vi "231124_Nikon_Control.vi"() -> ()   [LabVIEW 2025]
doc: "This simple VI control few elements of a Nikon Ti2 microscope.\nAny kind of supplementary element can be controlled with a new event type (flurorescence cube turret for example)"
uses:
  v2.1/SubVIS/Presets.ctl
panel:
  in  "Presets":T1=2 items=["1- Bino - Brightfield"=1, "2- Bino - Fluo"=2, "3- Right"=3, "4- Left"=4]
  in  "Cluster commandes":T2={"Dia lamp"=TRUE, "Dia lamp intensity"=1689.1304347826087, "Objective"=2, "Light path"=2, "Z pos (µm)"=335593} {"Z pos (µm)" min=0 max=990000 step=100 scale=0.0..990000.0; "Light path" items=["1- Eyepiece"=1, "2- Right"=2, "3- Left + Eyepiece"=3, "4- Left"=4]; "Objective" items=["1- Target"=1, "2- PLAN APO 100X 1,45 Oil"=2, "3- Empty"=3, "4- Empty"=4, "5- Empty"=5, "6- Empty"=6]; "Dia lamp intensity" scale=0.0..2100.0}
  out "Cluster µscope":T3
  in  "stop":bool
  in  "NikonTi2AxLib.INikonTi2AxMicroscope":refnum<k7>
  out "error out":errorcluster={"status"=TRUE, "code"=-9, "source"="Exception occured in Nikon.Ti2.Microscope.1: Failed in 231026_NikonTi2_Indicators_v2.vi"} caption="sortie d'erreur"
  in  "error in":errorcluster caption="entrée d'erreur"
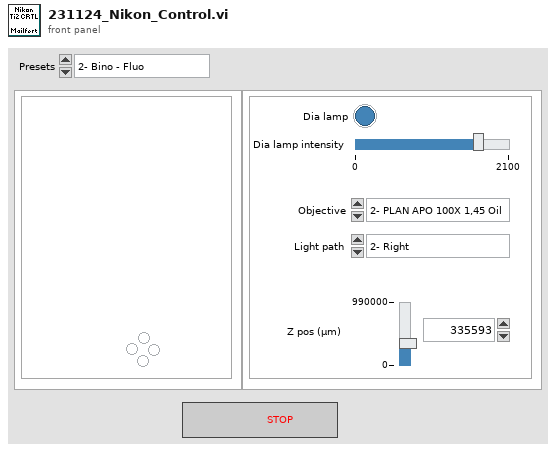
[diagram p1: front panel]
types:
  T1 = typedef "Presets.ctl" = u8
  T2 = cluster{"Dia lamp":bool, "Dia lamp intensity":dbl, "Objective":i32, "Light path":u32, "Z pos (µm)":i32}
  T3 = cluster{"Eyepiece":bool, "Right":bool, "Left + Eyepiece":bool, "Left":bool}
  T4 = cluster{"iNOSEPIECE":i32, "iLIGHTPATH":i32, "iDIA_LAMP_Switch":i32, "iDIA_LAMP_Pos":i32, "iZPOSITION":i32, "iPFS_SWITCH":i32, "iPFS_STATUS":i32, "iPFS_OFFSET":i32}
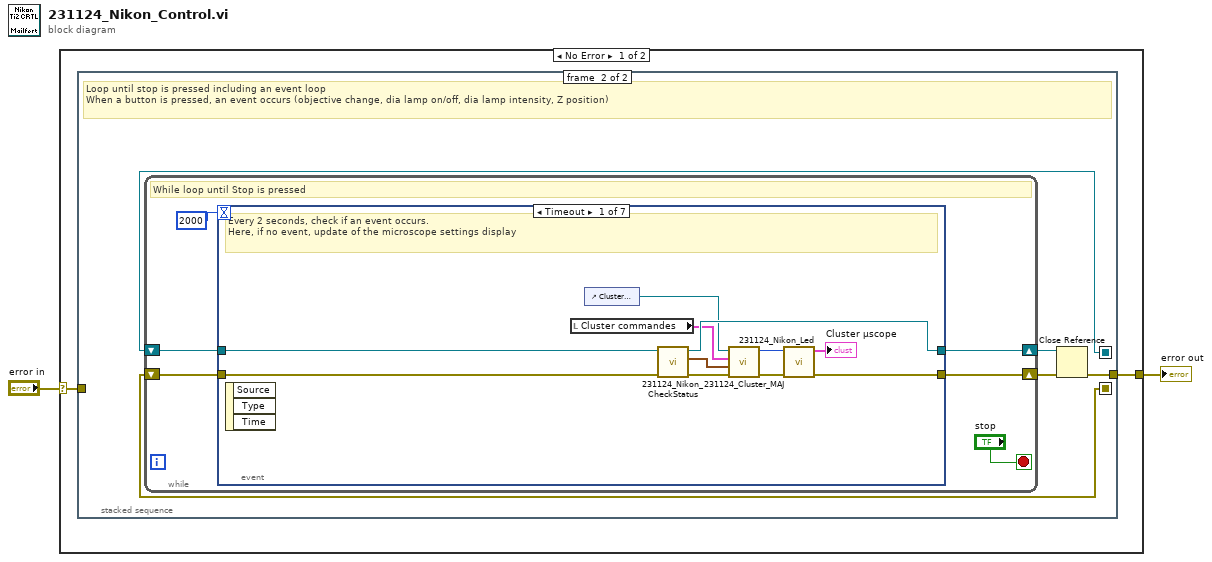
[diagram p0: block diagram]
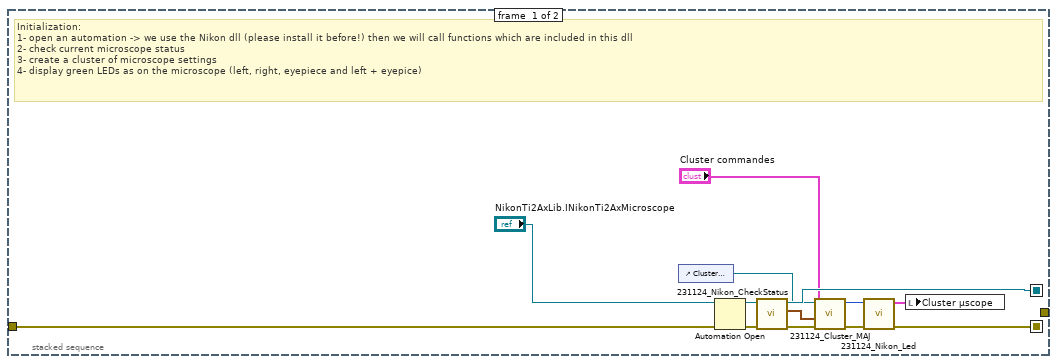
[diagram p2: hidden frame]
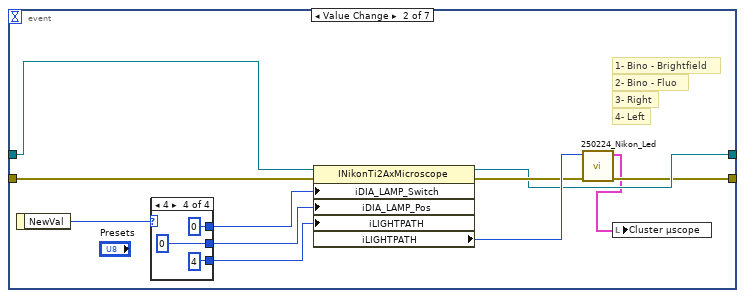
[diagram p3: hidden frame]
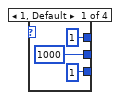
[diagram p4: hidden frame]
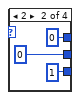
[diagram p5: hidden frame]
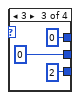
[diagram p6: hidden frame]
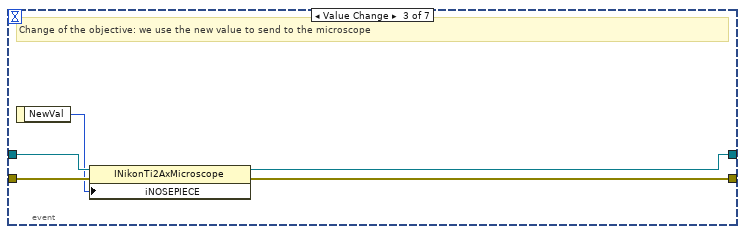
[diagram p7: hidden frame]
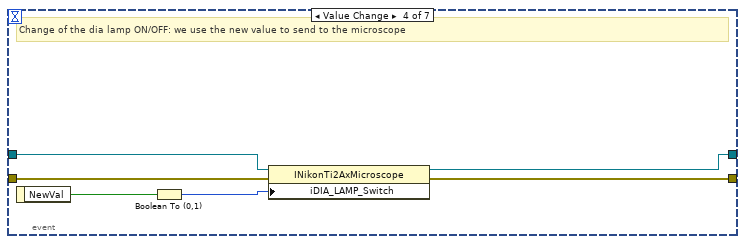
[diagram p8: hidden frame]
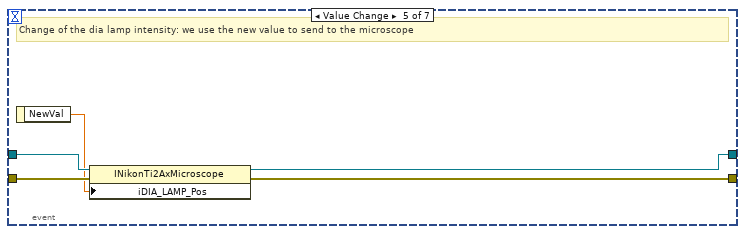
[diagram p9: hidden frame]
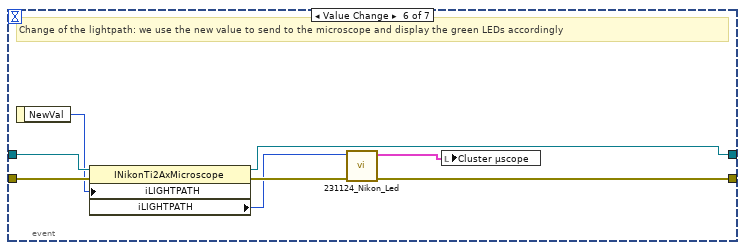
[diagram p10: hidden frame]
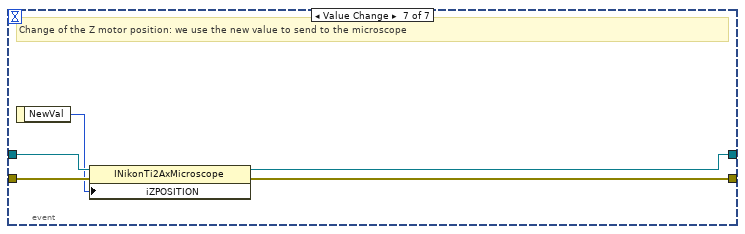
[diagram p11: hidden frame]
diagram:
  n1 = case shown="No Error" "error in" {
    selector: "error in" -> [w4 w92]
    tunnel: [w3 w92] -> w1
    frame No Error {
      n2 = stacked-sequence {
        seq-local: [w13 _] -> [_ w22]
        seq-local: [w6 _] -> [_ w18]
        tunnel: w4 -> [w14 _]
        tunnel: [_ w19] -> w3
        frame #0 {
          # "Initialization:\n1- open an automation -> we use the Nikon dll (please install it before!) then we will call functions which are included in this dll\n2- check current microscope status\n3- create a cluster of microscope settings\n4- display green LEDs as on the microscope (left, right, eyepiece and left + eyepice)"
          n3 = control-ref of="Cluster commandes"() -> (w5:refnum<vi>)
          n4 = Automation Open(error in (no error)=w14, Automation Refnum="NikonTi2AxLib.INikonTi2AxMicroscope") -> (Automation Refnum=w16:refnum<k7>, error out=w15:errorcluster)  [unwired: 2 in]
          n5 = call "231124_Nikon_CheckStatus.vi"("error in"=w15, "NikonTi2AxLib.INikonTi2AxMicroscope"=w16) -> ("error out"=w8:errorcluster, "Nikon status cluster"=w12:T4, "reference out"=w13:refnum<k7>)  [unwired: 7 in]
          n6 = call "231124_Cluster_MAJ.vi"("error in (no error)"=w8, "Nikon status cluster"=w12, 10:"Cluster commandes"="Cluster commandes", 11:"Cluster commandes"=w5) -> ("error out"=w7:errorcluster, "iLIGHTPATH"=w9:i32)  [unwired: 5 in, 1 out]
          n7 = call "231124_Nikon_Led.vi"("error in"=w7, "Light path"=w9) -> ("error out"=w6:errorcluster, "Cluster µscope"=w11:T3)  [unwired: 8 in]
          n8 = local write "Cluster µscope"(w11) -> ()
        }
        frame #1 {
          # "Loop until stop is pressed including an event loop\nWhen a button is pressed, an event occurs (objective change, dia lamp on/off, dia lamp intensity, Z position)"
          n9 = while {
            shift-right: [w23] -> w20
            shift-left: w18 -> [w28]
            shift-right: [w24] -> w21
            shift-left: w22 -> [w25]
            stop <- "stop" stop-if-true
            # "While loop until Stop is pressed"
            n10 = event shown="[0] Timeout" {
              selector: _ -> [_ _ _ _ _ _ _]
              dyn-events: _ -> [_ _ _ _ _ _ _]
              timeout: 2000 -> [_ _ _ _ _ _ _]
              tunnel: [w36 w42 w64 w70 w75 w83 w90] -> w23
              tunnel: w28 -> [w39 w41 w66 w72 w77 w84 w88]
              tunnel: w25 -> [w38 w44 w67 w73 w78 w85 w89]
              tunnel: [w37 w43 w65 w71 w76 w86 w91] -> w24
              event Timeout {
                # "Every 2 seconds, check if an event occurs.\nHere, if no event, update of the microscope settings display"
                n11 = event-data() -> ()  [unwired: 1 in, 3 out]
                n12 = local read "Cluster commandes"() -> (w30:T2)
                n13 = control-ref of="Cluster commandes"() -> (w29:refnum<vi>)
                n14 = call "231124_Nikon_CheckStatus.vi"("error in"=w39, "NikonTi2AxLib.INikonTi2AxMicroscope"=w38) -> ("error out"=w33:errorcluster, "Nikon status cluster"=w34:T4, "reference out"=w37:refnum<k7>)  [unwired: 7 in]
                n15 = call "231124_Cluster_MAJ.vi"("error in (no error)"=w33, "Nikon status cluster"=w34, 10:"Cluster commandes"=w30, 11:"Cluster commandes"=w29) -> ("error out"=w32:errorcluster, "iLIGHTPATH"=w31:i32)  [unwired: 5 in, 1 out]
                n16 = call "231124_Nikon_Led.vi"("error in"=w32, "Light path"=w31) -> ("error out"=w36:errorcluster, "Cluster µscope"=→"Cluster µscope":T3)  [unwired: 8 in]
              }
              event Value Change {
                # "1- Bino - Brightfield"
                # "4- Left"
                # "3- Right"
                # "2- Bino - Fluo"
                n17 = event-data() -> ("NewVal"=w45:T1)  [unwired: 1 in]
                n18 = case shown="4" w45 {
                  tunnel: [1 0 0 0] -> w48
                  tunnel: [1000 0 0 0] -> w49
                  tunnel: [1 ("iLIGHTPATH") 1 ("iLIGHTPATH") 2 ("iLIGHTPATH") 4 ("iLIGHTPATH")] -> w50
                  frame 1, Default {
                  }
                  frame 2 {
                  }
                  frame 3 {
                  }
                  frame 4 {
                  }
                }
                n19 = property class="INikonTi2AxMicroscope"(reference=w44, error in=w41, "iDIA_LAMP_Switch"=w48, "iDIA_LAMP_Pos"=w49, "iLIGHTPATH"=w50) -> (reference out=w43:refnum<k7>, error out=w46:errorcluster, "iLIGHTPATH"=w47:i32)
                n20 = call "250224_Nikon_Led.vi"("error in"=w46, "Light path"=w47) -> ("error out"=w42:errorcluster, "Cluster µscope"=w40:T3)  [unwired: 8 in]
                n21 = local write "Cluster µscope"(w40) -> ()
              }
              event "Cluster commandes.Objective": Value Change {
                # "Change of the objective: we use the new value to send to the microscope"
                n22 = event-data() -> ("NewVal"=w63:i32)  [unwired: 1 in]
                n23 = property class="INikonTi2AxMicroscope"(reference=w67, error in=w66, "iNOSEPIECE"=w63) -> (reference out=w65:refnum<k7>, error out=w64:errorcluster)
              }
              event "Cluster commandes.Dia lamp": Value Change {
                # "Change of the dia lamp ON/OFF: we use the new value to send to the microscope"
                n24 = event-data() -> ("NewVal"=w69:bool)  [unwired: 1 in]
                n25 = Boolean To (0,1)(Boolean=w69) -> (0, 1=w68:i16)
                n26 = property class="INikonTi2AxMicroscope"(reference=w73, error in=w72, "iDIA_LAMP_Switch"=w68) -> (reference out=w71:refnum<k7>, error out=w70:errorcluster)
              }
              event "Cluster commandes.Dia lamp intensity": Value Change {
                # "Change of the dia lamp intensity: we use the new value to send to the microscope"
                n27 = event-data() -> ("NewVal"=w74:dbl)  [unwired: 1 in]
                n28 = property class="INikonTi2AxMicroscope"(reference=w78, error in=w77, "iDIA_LAMP_Pos"=w74) -> (reference out=w76:refnum<k7>, error out=w75:errorcluster)
              }
              event "Cluster commandes.Light path": Value Change {
                # "Change of the lightpath: we use the new value to send to the microscope and display the green LEDs accordingly"
                n29 = event-data() -> ("NewVal"=w80:u32)  [unwired: 1 in]
                n30 = property class="INikonTi2AxMicroscope"(reference=w85, error in=w84, "iLIGHTPATH"=w80) -> (reference out=w86:refnum<k7>, error out=w82:errorcluster, "iLIGHTPATH"=w81:i32)
                n31 = call "231124_Nikon_Led.vi"("error in"=w82, "Light path"=w81) -> ("error out"=w83:errorcluster, "Cluster µscope"=w79:T3)  [unwired: 8 in]
                n32 = local write "Cluster µscope"(w79) -> ()
              }
              event "Cluster commandes.Z pos (µm)": Value Change {
                # "Change of the Z motor position: we use the new value to send to the microscope"
                n33 = event-data() -> ("NewVal"=w87:i32)  [unwired: 1 in]
                n34 = property class="INikonTi2AxMicroscope"(reference=w89, error in=w88, "iZPOSITION"=w87) -> (reference out=w91:refnum<k7>, error out=w90:errorcluster)
              }
            }
          }
          n35 = Close Reference(reference=w21, error in (no error)=w20) -> (error out=w19:errorcluster)
        }
      }
    }
    frame Error {
    }
  }
  "error out" <- w1
